vi "Client Get Enum Value from Proto Value.vi"(8 "error in (no error)":errorcluster, 9 "value in proto":i32, 10 "enum name":string, 11 "gRPC ID in":T1) -> (0 "error out":errorcluster, 2 "value in LV":u32, 3 "gRPC ID out":T1)   [LabVIEW 2024, in "grpc-lvsupport.lvlib"]
uses:
  grpc-lvsupport.lvlib
  grpcId.ctl
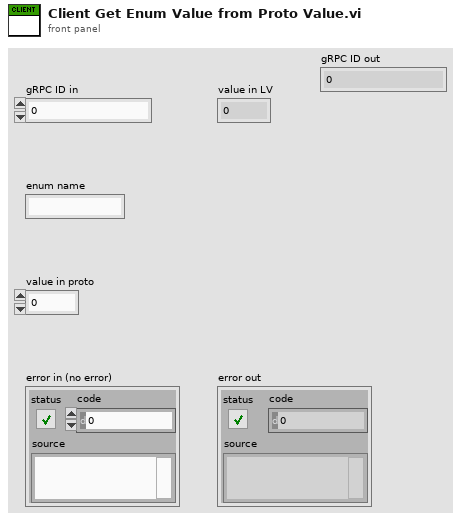
[diagram p1: front panel]
types:
  T1 = typedef "grpc-lvsupport.lvlib/grpcId.ctl" = u64
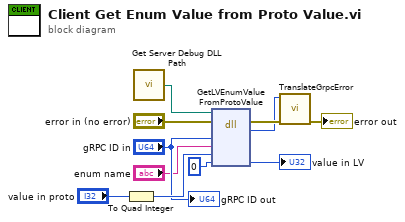
[diagram p0: block diagram]
diagram:
  n1 = To Quad Integer(1:"value in proto") -> (0:w11:i64)
  n2 = call "Get Server Debug DLL Path.vi"() -> ("DLL Path"=w9:path)
  n3 = dll-call lib="?" fn="GetLVEnumValueFromProtoValue"(path in=w9, error in="error in (no error)", "gRPC ID in"="gRPC ID in", "enum name"="enum name", "value in proto"=w11, "value in LV"=u32 0) -> (error out=w7:errorcluster, "error code"=w6:i32, "value in LV"=→"value in LV":u32)  [unwired: 4 in, 1 out]
  n4 = call "TranslateGrpcError.vi"("error in"=w7, "Error Code"=w6) -> ("error out"=→"error out":errorcluster)  [unwired: 9 in]
  "gRPC ID out" <- "gRPC ID in"
